vi "Send RegisterForMessageSpecificType.vi"(7 "Message Priority (Normal)":T1=enum."Normal", 8 "error in (no error)":errorcluster, 9 "Message Enqueuer 2":refnum<class "Message Enqueuer.lvclass">, 10 "MailBoxMessage":refnum<class "MailBoxMessage.lvclass">, 11 "Message Enqueuer":refnum<class "Message Enqueuer.lvclass">) -> (0 "error out":errorcluster, 3 "Message Enqueuer out":refnum<class "Message Enqueuer.lvclass">)   [LabVIEW 2020, in "MailboxManager.lvlib" / "RegisterForMessageSpecificType Msg.lvclass"]
doc: "This VI sends the message to an actor."
uses:
  RegisterForMessageSpecificType Msg.lvclass
  <vilib>/ActorFramework/Message Enqueuer/Message Enqueuer.lvclass
  <vilib>/ActorFramework/Message Enqueuer/Message Priority.ctl
  C:/Program Files (x86)/National Instruments/LabVIEW 2020/vi.lib/ActorFramework/Message/Message.lvclass
  RegisterForMessageSpecificType Msg.lvclass/RegisterForMessageSpecificType Msg.ctl
  <vilib>/ActorFramework/Message Enqueuer/Message Enqueuer.lvclass/Message Enqueuer.ctl
  <vilib>/ActorFramework/Message Priority Queue/Priority Enqueue.vi
  C:/Users/taylo/Projects/LabVIEW/ActorMailbox/MailboxManager/MailboxManager Messages/RegisterForMessageSpecificType Msg/RegisterForMessageSpecificType Msg.lvclass
  MailBoxMessage/MailBoxMessage.lvclass
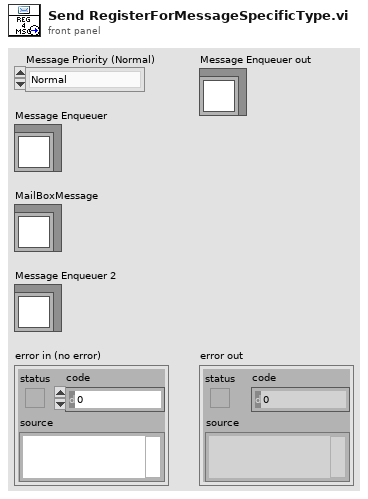
[diagram p1: front panel]
types:
  T1 = typedef "Actor Framework.lvlib/Message Enqueuer.lvclass/Message Priority.ctl" = enum16{"Low", "Normal", "High"}
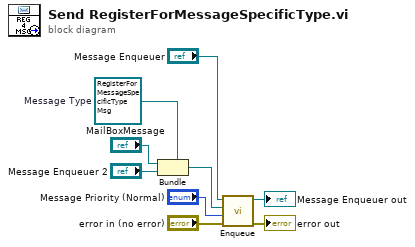
[diagram p0: block diagram]
diagram:
  w6 = refnum<class "RegisterForMessageSpecificType Msg.lvclass"> refnum  # Message Type
  n1 = Bundle(cluster=w6, "MailBoxMessage", "Message Enqueuer 2") -> (w5:refnum<class "RegisterForMessageSpecificType Msg.lvclass">)
  n2 = call <vilib>:"Enqueue.vi"("error in (no error)"="error in (no error)", "Message Priority (Normal)"="Message Priority (Normal)", "Message"=w5, "Message Enqueuer in"="Message Enqueuer") -> ("error out"=→"error out":errorcluster, "Message Enqueuer out"=→"Message Enqueuer out":refnum<class "Message Enqueuer.lvclass">)  [unwired: 6 in]
